vi "Test Bench v17 - TDMS - NOTWORKING.vi"() -> ()   [LabVIEW 2022 SP3]
uses:
  WhiteNoise.ctl
  <vilib>/Utility/error.llb/DialogType.ctl
  <vilib>/Platform/TimedLoop/XDataNode/timing_clust.ctl
  <vilib>/Platform/TimedLoop/XDataNode/nitl_modes.ctl
  <vilib>/Platform/TimedLoop/XDataNode/wakeup.ctl
  <vilib>/DAQmx/write.llb/DAQmx Write (Analog 2D DBL NChan NSamp).vi
  <vilib>/DAQmx/read.llb/DAQmx Read (Analog 1D DBL 1Chan NSamp).vi
  <vilib>/DAQmx/create/channels.llb/DAQmx Create Channel (AI-Acceleration-Accelerometer).vi
  <vilib>/DAQmx/create/channels.llb/DAQmx Create Channel (AO-Voltage-Basic).vi
  <vilib>/DAQmx/configure/timing.llb/DAQmx Timing (Sample Clock).vi
  <vilib>/DAQmx/miscellaneous.llb/DAQmx Fill In Error Info.vi
  <vilib>/platform/TimedLoop/XDataNode/XDataNode.xnode
  <resource>/objmgr/daqmx.rc
  <vilib>/measure/NI_MABase.lvlib
  <vilib>/Platform/TimedLoop/XDataNode/XDNodeRunTimeDep.lvlib
panel:
  out "TotalSampPerChanAcquired":dbl
  in  "stop":bool
  out "SampClk.Rate":dbl
  out "Accel. 1 Raw":dbl[](graph)
  in  "Enable Display":bool=TRUE
  in  "Folder to save file to":path=path "C:/Users/LAV-UFSC-2023/Documents/LAV-TCC/Dados-Experimentos/Dados-Bancada-LABVIEW"
  out "Output Signal":dynamicdata(graph)
  in  "Accel. 2":bool
  out "New file path":path
  in  "Signal Output\nControl":enum32{"White Noise", "Harmonic"}(tab)
  in  "White Noise\nParameters":T2={"Seed"=0.0, "Standard Deviation"=0.2, "Reset"=FALSE, "Iterator"=1.0, "Seed"=-1, "Lower Cut-Off"=5.0, "Upper Cut-Off"=350.0} {"Upper Cut-Off" min=5.0 max=350.0 step=10.0; "Lower Cut-Off" min=5.0 max=350.0 step=10.0; "Standard Deviation" min=0.001 max=3.0 step=0.05 format="%0.2p"}
  out "dt White Noise":dbl
  in  "Hamonic\nParameters":T3={"Waveform Type"=0, "Frequency"=10.0, "Amplitude"=0.25} {"Frequency" min=5.0 max=350.0 step=10.0 format="%0.2p"; "Waveform Type" items=["Sine Wave", "Triangle Wave", "Square Wave", "Sawtooth Wave"]; "Amplitude" min=0.001 max=0.3 step=0.05 format="%0.2p"}
  out "dt Harmonic":dbl
  in  "Output":bool=TRUE
  # "Filter"
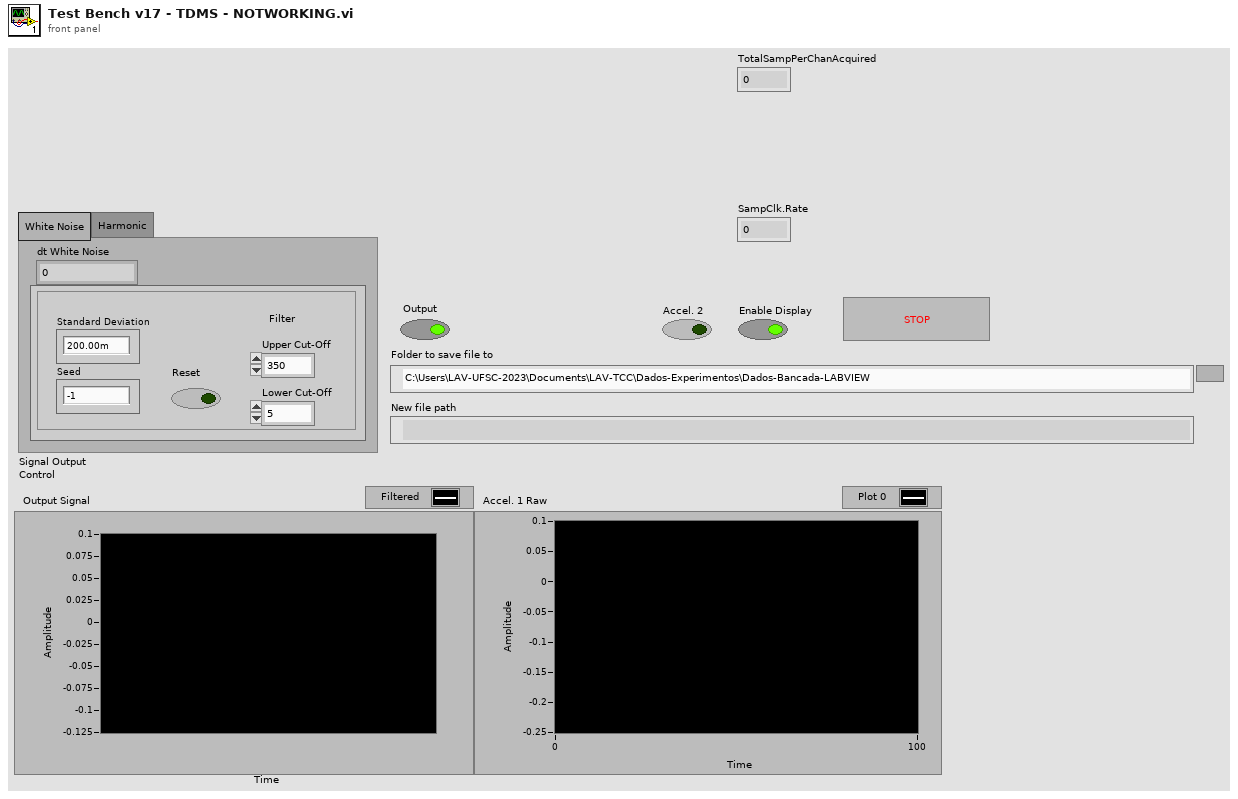
[diagram p1: front panel]
types:
  T1 = typedef "WhiteNoise.ctl" = dbl
  T2 = cluster{"Seed":T1, "Standard Deviation":dbl, "Reset":bool, "Iterator":dbl, "Seed":i8, "Lower Cut-Off":dbl, "Upper Cut-Off":dbl}
  T3 = cluster{"Waveform Type":u16, "Frequency":dbl, "Amplitude":dbl}
  T4 = typedef "DialogType.ctl" = u16
  T5 = enum16{"open", "open or create", "create or replace", "create", "open (read-only)"}
  T6 = typedef "XDNodeRunTimeDep.lvlib/timing_clust.ctl" = cluster{"Expected End [f-1]":u64, "Actual End [f-1]":u64, "Finished Late? [f-1]":bool, "Expected End [i-1]":u64, "Actual End [i-1]":u64, "Finished Late? [i-1]":bool, "Expected Start [i]":u64, "Actual Start [i]":u64, "Expected Start [f]":u64, "Actual Start [f]":u64, "Source Name":string, "Structure Name":string, "Period":i64, "Deadline":i64, "Offset":i64, "Start":i64, "Priority":i32, "Timeout":i32, "Mode":T7, "Wakeup Reason":T8, "Error":errorcluster, "Source Type":string, "Secondary Source Type":string, "Global End Time":u64, "Global Start Time":u64, "Frame Duration":u64, "Iteration Duration":u64, "Assigned CPU":i32, "I/O Scan Engine Mode":u32}
  T7 = typedef "XDNodeRunTimeDep.lvlib/nitl_modes.ctl" = enum32{"No Change", "Process missed periods, maintain original phase", "Discard missed periods, maintain original phase", "Process missed periods, ignore original phase", "Discard missed periods, ignore original phase"}
  T8 = typedef "XDNodeRunTimeDep.lvlib/wakeup.ctl" = enum32{"Normal", "Aborted", "Asynchronous wakeup", "Timing source error", "Timed loop error", "Timeout"}
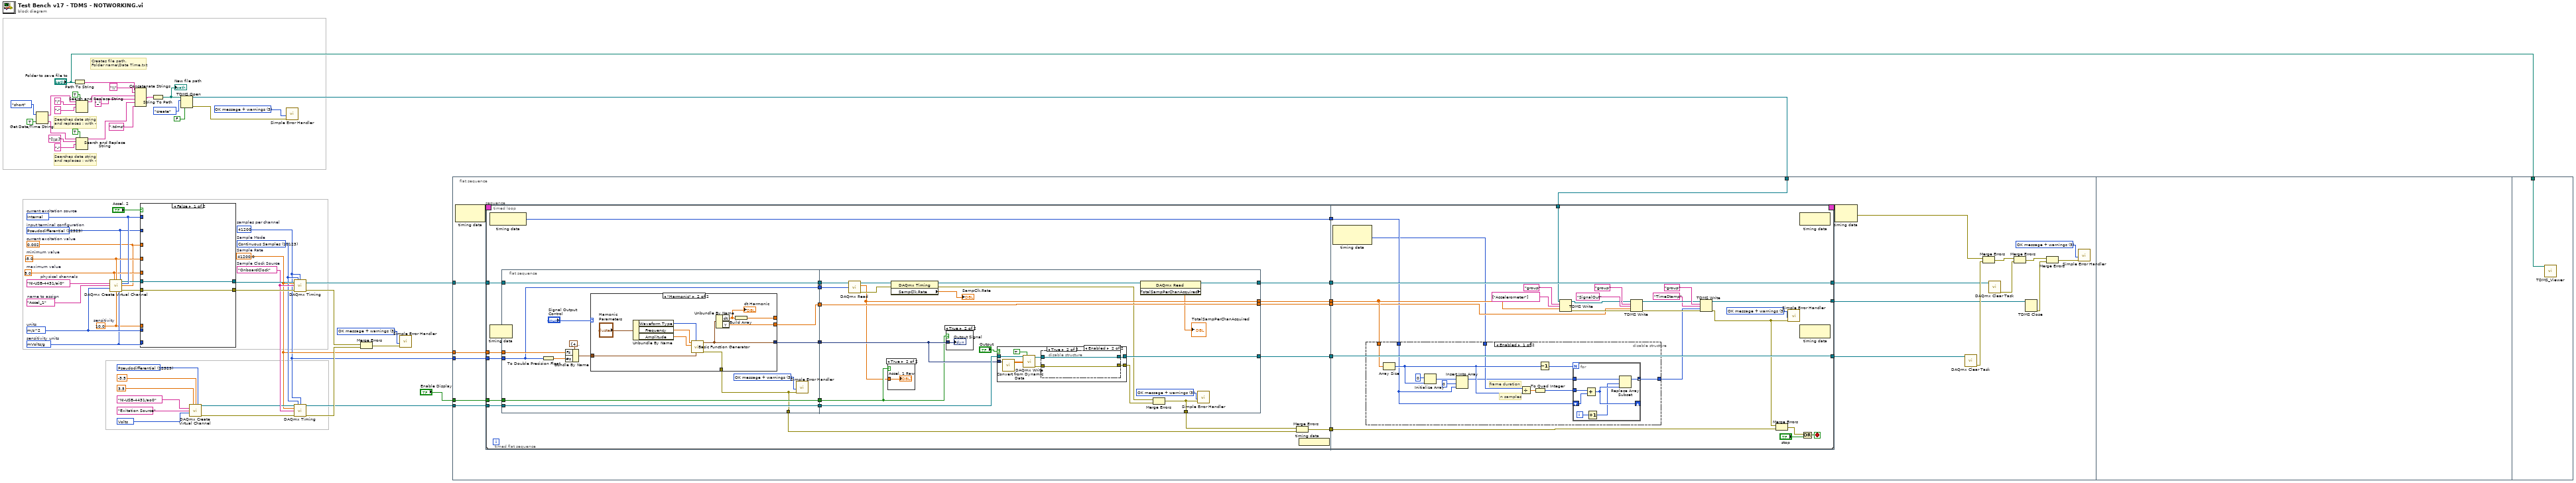
[diagram p0: block diagram]
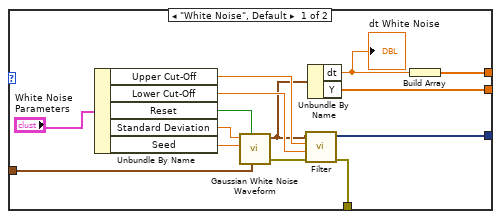
[diagram p2: hidden frame]
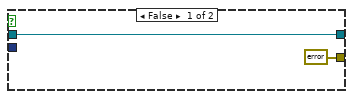
[diagram p5: hidden frame]
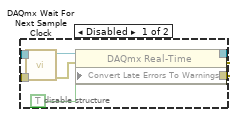
[diagram p6: hidden frame]
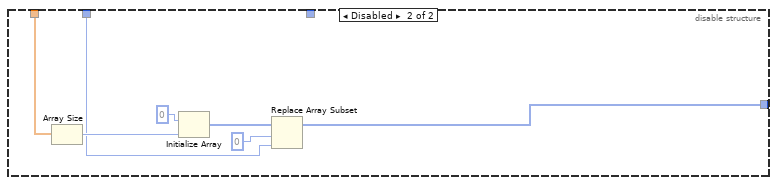
[diagram p7: hidden frame]
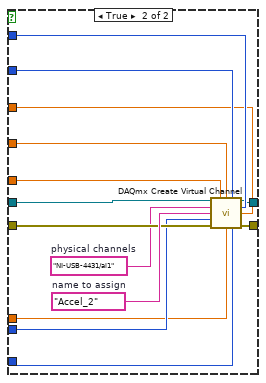
[diagram p8: hidden frame]
diagram:
  w10 = T4 3 items=["no dialog", "OK message", "continue or stop message", "OK message + warnings", "continue/stop + warnings"] ("type of dialog (OK msg:1)")
  w6 = 41200  # samples per channel
  w12 = T4 3 items=["no dialog", "OK message", "continue or stop message", "OK message + warnings", "continue/stop + warnings"] ("type of dialog (OK msg:1)")
  w45 = 12529 items=["Default"=-1, "RSE"=10083, "Differential"=10106, "Pseudodifferential"=12529] ("output terminal configuration")
  w43 = 10348 items=["Volts"=10348, "From Custom Scale"=10065] ("units")
  w49 = 12509 items=["mVolts/g"=12509, "Volts/g"=12510]  # sensitivity units
  w40 = 10.0  # sensitivity
  w48 = 0.002  # current excitation value
  w56 = 10200 items=["Internal"=10200, "External"=10167, "None"=10230]  # current excitation source
  w50 = tag "NI-USB-4431/ai0"  # physical channels
  w37 = tag "OnboardClock"  # Sample Clock Source
  w7 = 41200.0  # Sample Rate
  w36 = 10123 items=["Finite Samples"=10178, "Continuous Samples"=10123, "Hardware Timed Single Point"=12522]  # Sample Mode
  w52 = 12529 items=["default"=-1, "RSE"=10083, "NRSE"=10078, "Differential"=10106, "Pseudodifferential"=12529]  # input terminal configuration
  w55 = -5.0  # minimum value
  w54 = 5.0  # maximum value
  w58 = "Accel_1"  # name to assign
  w53 = 12470 items=["g"=10186, "m/s^2"=12470, "in/s^2"=12471, "From Custom Scale"=10065]  # units
  # "Searches date string\nand replaces : with -"
  # "Searches date string\nand replaces : with -"
  # "Creates file path.\nFolder name\\Date Time.txt"
  n1 = Get Date/Time String(date format (0)=enum16{"short", "long", "abbreviated"}."short", want seconds? (F)=TRUE) -> (date string=w15:string, time string=w28:string)  [unwired: 1 in]
  n2 = Path To String(path="Folder to save file to") -> (string=w23:string)
  n3 = Search and Replace String(replace all?=TRUE ("replace all? (F)"), input string=w15, search string="/" ("replace string (\"\")"), replace string="-" ("replace string (\"\")")) -> (result string=w14:string)  [unwired: 4 in, 3 out]
  n4 = Search and Replace String(replace all?=TRUE ("replace all? (F)"), input string=w28, search string="[\\s:]" ("replace string (\"\")"), replace string="-" ("replace string (\"\")")) -> (result string=w21:string)  [unwired: 4 in, 3 out]
  n5 = call-poly <vilib>:"DAQmx Create Virtual Channel.vi"("maximum value"=w54, "minimum value"=w55, "input terminal configuration"=w52, "physical channels"=w50, "current excitation source"=w56, "name to assign"=w58, "current excitation value"=w48, "units"=w53, "sensitivity"=w40, "sensitivity units"=w49) -> ("task out"=w51:refnum<k21>, "error out"=w57:errorcluster)  [unwired: 4 in]
  n6 = Concatenate Strings(w23, "\\" ("string"), w14, "_" ("string"), w21, ".tdms" ("string")) -> (w19:string)
  n7 = case shown="False" "Accel. 2" {
    tunnel: w57 -> [w60 w73]
    tunnel: w56 -> [_ w72]
    tunnel: w55 -> [_ w71]
    tunnel: w54 -> [_ w70]
    tunnel: w53 -> [_ w69]
    tunnel: w52 -> [_ w68]
    tunnel: w51 -> [w59 w67]
    tunnel: w49 -> [_ w65]
    tunnel: w48 -> [_ w64]
    tunnel: w40 -> [_ w63]
    tunnel: [w60 w62] -> w39
    tunnel: [w59 w61] -> w38
    frame False {
    }
    frame True {
      w66 = tag "NI-USB-4431/ai1"  # physical channels
      w74 = "Accel_2"  # name to assign
      n8 = call-poly <vilib>:"DAQmx Create Virtual Channel.vi"("task in"=w67, "maximum value"=w70, "minimum value"=w71, "input terminal configuration"=w68, "physical channels"=w66, "current excitation source"=w72, "name to assign"=w74, "current excitation value"=w64, "units"=w69, "error in"=w73, "sensitivity"=w63, "sensitivity units"=w65) -> ("task out"=w61:refnum<k21>, "error out"=w62:errorcluster)  [unwired: 2 in]
    }
  }
  n9 = String To Path(string=w19) -> (path=w5:path)
  "New file path" <- w5
  n10 = TDMS Open(6:FALSE ("enable asynchronous? (T)"), 10:T5."create" ("operation (0:open)"), 11:w5) -> (0:w1:errorcluster, 3:w2:refnum<k34>)  [unwired: 4 in]
  n11 = call-poly <vilib>:"DAQmx Create Virtual Channel.vi"("maximum value"=3.5, "minimum value"=-3.5, "output terminal configuration"=w45, "physical channels"=tag "NI-USB-4431/ao0", "name to assign"="Exitation Source", "units"=w43) -> ("task out"=w34:refnum<k21>, "error out"=w35:errorcluster)  [unwired: 8 in]
  n12 = call <vilib>:"Simple Error Handler.vi"("type of dialog (OK msg:1)"=w12, "error in (no error)"=w1) -> ()  [unwired: 3 in, 5 out]
  n13 = call-poly <vilib>:"DAQmx Timing.vi"("task/channels in"=w38, "sample mode"=w36, "samples per channel"=w6, "rate"=w7, "source"=w37, "error in"=w39) -> ("task out"=w9:refnum<k21>, "error out"=w42:errorcluster)  [unwired: 8 in]
  n14 = call-poly <vilib>:"DAQmx Timing.vi"("task/channels in"=w34, "sample mode"=w36, "samples per channel"=w6, "rate"=w7, "source"=w37, "error in"=w35) -> ("task out"=w32:refnum<k21>, "error out"=w33:errorcluster)  [unwired: 8 in]
  n15 = Merge Errors(w42, w33) -> (w8:errorcluster)
  n16 = call <vilib>:"Simple Error Handler.vi"("type of dialog (OK msg:1)"=w10, "error in (no error)"=w8) -> ()  [unwired: 3 in, 5 out]
  n17 = flat-sequence {
    tunnel: w32 -> [w90]
    tunnel: w9 -> [w88]
    tunnel: w2 -> [w80]
    tunnel: "Enable Display" -> [w87]
    tunnel: w7 -> [w79]
    tunnel: w6 -> [w78]
    tunnel: "Folder to save file to" -> [w276]
    frame #0 {
      w91 = T4 3 items=["no dialog", "OK message", "continue or stop message", "OK message + warnings", "continue/stop + warnings"] ("type of dialog (OK msg:1)")
      n18 = node-c288() -> (w93:T6)  [unwired: 1 in]
      n19 = timed-loop {
        tunnel: w90 -> [w102]
        tunnel: [w101] -> w89
        tunnel: w88 -> [w100]
        tunnel: [w96] -> w85
        tunnel: [w94] -> w77
        tunnel: w87 -> [w99]
        tunnel: w78 -> [w98]
        timing: w93 -> [_]
        timing-out: [_] -> w92
        tunnel: w80 -> [w97]
        tunnel: w79 -> [w95]
        stop <- w237 stop-if-true
        n20 = timed-sequence {
          timing: _ -> [_]
          timing-out: _ -> [_]
          tunnel: w102 -> [w117]
          tunnel: [w116] -> w101
          tunnel: w100 -> [w115]
          tunnel: w99 -> [w114]
          tunnel: w98 -> [w113]
          tunnel: w97 -> [w109]
          tunnel: [w108] -> w96
          tunnel: w95 -> [w105]
          tunnel: [w104] -> w94
          n21 = timed-flat-sequence {
            tunnel: w117 -> [w130]
            tunnel: w115 -> [w129]
            tunnel: w114 -> [w126]
            tunnel: w113 -> [w125]
            tunnel: [w128] -> w112
            tunnel: [w127] -> w111
            tunnel: [w122] -> w110
            tunnel: [w121] -> w107
            tunnel: [w120] -> w106
            tunnel: w105 -> [w119]
            tunnel: [w118] -> w103
            tunnel: [w241] -> w116
            tunnel: w112 -> [w241]
            tunnel: w111 -> [w235]
            tunnel: w110 -> [w238]
            tunnel: w109 -> [w224]
            tunnel: [w235] -> w108
            tunnel: w107 -> [w233]
            tunnel: w106 -> [w225]
            tunnel: [w229] -> w104
            tunnel: w103 -> [w218]
            frame #0 {
              n22 = node-c288() -> (w118:i64)  [unwired: 1 in]
              n23 = flat-sequence {
                tunnel: [w149] -> w136
                tunnel: [w145] -> w135
                tunnel: [w148] -> w134
                tunnel: [w146] -> w133
                tunnel: [w147] -> w132
                tunnel: [w141] -> w131
                tunnel: [w144] -> w123
                tunnel: w130 -> [w148]
                tunnel: w129 -> [w149]
                tunnel: w126 -> [w146]
                tunnel: w125 -> [w141]
                tunnel: w119 -> [w142]
                tunnel: w136 -> [w187]
                tunnel: w135 -> [w195]
                tunnel: w134 -> [w193]
                tunnel: w133 -> [w188]
                tunnel: w132 -> [w191]
                tunnel: w131 -> [w186]
                tunnel: [w180] -> w124
                tunnel: [w184] -> w121
                tunnel: [w195] -> w120
                tunnel: [w192] -> w128
                tunnel: [w179] -> w127
                frame #0 {
                  w143 = T4 3 items=["no dialog", "OK message", "continue or stop message", "OK message + warnings", "continue/stop + warnings"] ("type of dialog (OK msg:1)")
                  n24 = To Double Precision Float(number=w141) -> (double precision float=w140:dbl)
                  n25 = Bundle By Name(cluster=cluster{"Fs":dbl, "#s":dbl} {"Fs"=41200.0, "#s"=41200.0} ("sampling info"), "Fs"=w142, "#s"=w140) -> (w151:cluster{"Fs":dbl, "#s":dbl})
                  n26 = case shown="\"Harmonic\"" "Signal Output\nControl" {
                    tunnel: w151 -> [w164 w175]
                    tunnel: [w156 w170] -> _
                    tunnel: [w155 w169] -> w147
                    tunnel: [w154 w168] -> w145
                    tunnel: [w153 w167] -> w144
                    frame "White Noise", Default {
                      n27 = Unbundle By Name("White Noise\nParameters") -> ("Upper Cut-Off"=w160:dbl, "Lower Cut-Off"=w159:dbl, "Reset"=w161:bool, "Standard Deviation"=w162:dbl, "Seed"=w163:T1)
                      n28 = call <vilib>:"Gaussian White Noise Waveform.vi"("sampling info"=w164, "reset signal"=w161, "seed"=w163, "standard deviation"=w162) -> ("error out"=w166:errorcluster, "signal out"=w158:waveform(dbl))  [unwired: 6 in]
                      n29 = call "Filter"("error in (no error)"=w166, "Lower Cut-Off"=w159, "Upper Cut-Off"=w160, "Signal"=w158) -> ("error out"=w153:errorcluster, "Filtered Signal"=w155:dynamicdata)  [unwired: 6 in]
                      n30 = Unbundle By Name(w158) -> ("dt"=w157:dbl, "Y"=w154:dbl[])
                      "dt White Noise" <- w157
                      n31 = Build Array(w157) -> (w156:dbl[])
                    }
                    frame "Harmonic" {
                      n32 = Unbundle By Name("Hamonic\nParameters") -> ("Waveform Type"=w174:u16, "Frequency"=w173:dbl, "Amplitude"=w172:dbl)
                      n33 = call <vilib>:"Basic Function Generator.vi"("sampling info"=w175, "signal type"=w174, "amplitude"=w172, "frequency"=w173) -> ("error out"=w167:errorcluster, "signal out"=w169:waveform(dbl))  [unwired: 5 in, 1 out]
                      n34 = Unbundle By Name(w169) -> ("dt"=w171:dbl, "Y"=w168:dbl[])
                      "dt Harmonic" <- w171
                      n35 = Build Array(w171) -> (w170:dbl[])
                    }
                  }
                  n36 = call <vilib>:"Simple Error Handler.vi"("type of dialog (OK msg:1)"=w143, "error in (no error)"=w144) -> ()  [unwired: 3 in, 5 out]
                }
                frame #1 {
                  w183 = T4 3 items=["no dialog", "OK message", "continue or stop message", "OK message + warnings", "continue/stop + warnings"] ("type of dialog (OK msg:1)")
                  n37 = call-poly <vilib>:"DAQmx Read.vi"("task/channels in"=w187, "number of samples per channel"=w186) -> ("task out"=w189:refnum<k21>, "data"=w184:dbl[], "error out"=w190:errorcluster)  [unwired: 11 in]
                  n38 = case shown="True" w188 {
                    tunnel: w184 -> [_ w196]
                    frame False {
                    }
                    frame True {
                      "Accel. 1 Raw" <- w196
                    }
                  }
                  n39 = property class="DAQmx Timing"(reference=w189, error in=w190) -> (reference out=w178:refnum<k21>, error out=w182:errorcluster, "SampClk.Rate"=→"SampClk.Rate":dbl)
                  n40 = case shown="True" w188 {
                    tunnel: w191 -> [_ w197]
                    frame False {
                    }
                    frame True {
                      "Output Signal" <- w197
                    }
                  }
                  n41 = case shown="True" "Output" {
                    tunnel: w193 -> [w199 w207]
                    tunnel: [errorcluster {"status"=FALSE, "code"=0, "source"=""} ("error out") w203] -> w181
                    tunnel: [w199 w204] -> w192
                    tunnel: w191 -> [_ w202]
                    frame False {
                    }
                    frame True {
                      n42 = call "Convert from Dynamic Data"("Dynamic Data Type"=w202) -> ("Array"=w201:dbl[][])  [unwired: 3 in]
                      n43 = call-poly <vilib>:"DAQmx Write.vi"("task/channels in"=w207, "auto start"=TRUE, "data"=w201) -> ("task out"=w206:refnum<k21>, "error out"=w205:errorcluster)  [unwired: 10 in, 1 out]
                      n44 = disable-structure shown="Enabled" {
                        disable-tunnel: w206 -> [w214 w215]
                        disable-tunnel: w205 -> [w213 w216]
                        disable-tunnel: [w211 w215] -> w204
                        disable-tunnel: [w210 w216] -> w203
                        frame Disabled {
                          n45 = call <vilib>:"DAQmx Wait For Next Sample Clock.vi"("task/channels in"=w214, "error in"=w213) -> ("task out"=w212:refnum<k21>, "error out"=w209:errorcluster)  [unwired: 11 in, 1 out]
                          n46 = property class="DAQmx Real-Time"(reference=w212, error in=w209, "Convert Late Errors To Warnings"=TRUE ("ConvLateErrorsToWarnings")) -> (reference out=w211:refnum<k21>, error out=w210:errorcluster)
                        }
                        frame Enabled {
                        }
                      }
                    }
                  }
                  n47 = property class="DAQmx Read"(reference=w178) -> (reference out=w179:refnum<k21>, "TotalSampPerChanAcquired"=→"TotalSampPerChanAcquired":dbl)  [unwired: 1 in, 1 out]
                  n48 = Merge Errors(w182, w181) -> (w180:errorcluster)
                  n49 = call <vilib>:"Simple Error Handler.vi"("type of dialog (OK msg:1)"=w183, "error in (no error)"=w180) -> ()  [unwired: 3 in, 5 out]
                }
              }
              n50 = Merge Errors(w124, w123) -> (w122:errorcluster)
              n51 = node-c288() -> ()  [unwired: 1 out]
            }
            frame #1 {
              w236 = T4 3 items=["no dialog", "OK message", "continue or stop message", "OK message + warnings", "continue/stop + warnings"] ("type of dialog (OK msg:1)")
              n52 = node-c288() -> (w217:i64)  [unwired: 1 in, 1 out]
              n53 = disable-structure shown="Enabled" {
                disable-tunnel: w233 -> [w253 w267]
                disable-tunnel: [w252 w264] -> w219
                disable-tunnel: w218 -> [w242 w261]
                disable-tunnel: w217 -> [w245 _]
                frame Enabled {
                  # "n samples"
                  # "frame duration"
                  n54 = Array Size(array=w253) -> (size(s)=w247:i32)
                  n55 = Initialize Array(i64 0, w247) -> (w249:i64[])
                  n56 = Insert Into Array(array=w249, index=0, new element=w242) -> (w244:i64[])
                  n57 = Divide(x=w245, y=w247) -> (x/y=w248:dbl)
                  n58 = To Quad Integer(1:w248) -> (0:w243:i64)
                  n59 = Decrement(x=w247) -> (x-1=w246:i32)
                  n60 = for {
                    N: w246 -> [_]
                    shift-right: [w258] -> _
                    shift-left: w242 -> [w257]
                    tunnel: w244 -> [w260]
                    tunnel: [w259] -> w252 mode=concatenating
                    tunnel: w243 -> [w254]
                    i -> [w256]
                    n61 = Add(x=w254, y=w257) -> (x+y=w258:i64)
                    n62 = Increment(x=w256) -> (x+1=w255:i32)
                    n63 = Replace Array Subset(array=w260, new element=w258, index=w255) -> (w259:i64[])
                  }
                }
                frame Disabled {
                  n64 = Array Size(array=w267) -> (size(s)=w262:i32)
                  n65 = Initialize Array(i64 0, w262) -> (w266:i64[])
                  n66 = Replace Array Subset(array=w266, new element=w261, index=0) -> (w264:i64[])
                }
              }
              n67 = TDMS Write(0:w224, 5:"group" ("group name in (Untitled)"), 7:string[] ["Accelerometer"] ("channel name(s) in (Untitled)"), 9:w233) -> (4:w223:refnum<k34>, 15:w227:errorcluster)  [unwired: 2 in, 2 out]
              n68 = TDMS Write(0:w223, 5:"group" ("group name in (Untitled)"), 7:"SignalOut", 9:w225, 11:w227) -> (4:w222:refnum<k34>, 15:w226:errorcluster)  [unwired: 1 in, 2 out]
              n69 = TDMS Write(0:w222, 5:"group" ("group name in (Untitled)"), 7:"TimeStamp", 9:w219, 11:w226) -> (4:w229:refnum<k34>, 15:w221:errorcluster)  [unwired: 1 in, 2 out]
              n70 = Merge Errors(w221, w238) -> (w240:errorcluster)
              n71 = call <vilib>:"Simple Error Handler.vi"("type of dialog (OK msg:1)"=w236, "error in (no error)"=w221) -> ()  [unwired: 3 in, 5 out]
              n72 = node-c288() -> ()  [unwired: 1 in, 1 out]
              n73 = Or(x=w240, y="stop") -> (x .or. y?=w237:bool)
            }
          }
        }
        n74 = node-c288() -> ()  [unwired: 1 in, 1 out]
        n75 = node-c288() -> ()  [unwired: 1 in, 1 out]
      }
      n76 = node-c288(w92) -> (w81:errorcluster)
      n77 = call <vilib>:"DAQmx Clear Task.vi"("task in"=w89) -> ("error out"=w86:errorcluster)  [unwired: 14 in]
      n78 = Merge Errors(w81, w86) -> (w84:errorcluster)
      n79 = call <vilib>:"DAQmx Clear Task.vi"("task in"=w85) -> ("error out"=w83:errorcluster)  [unwired: 14 in]
      n80 = Merge Errors(w84, w83) -> (w76:errorcluster)
      n81 = TDMS Close(11:w77) -> (0:w75:errorcluster)  [unwired: 1 in, 1 out]
      n82 = Merge Errors(w76, w75) -> (w82:errorcluster)
      n83 = call <vilib>:"Simple Error Handler.vi"("type of dialog (OK msg:1)"=w91, "error in (no error)"=w82) -> ()  [unwired: 3 in, 5 out]
    }
    frame #1 {
    }
    frame #2 {
      n84 = call "TDMS_Viewer.vi"("Data Directory"=w276) -> ()  [unwired: 11 in]
    }
  }
